vi "SaveIniRegExtSession.vi"(8 "error in (no error)":errorcluster, 11 "RegExt":T1) -> (0 "error out":errorcluster)   [LabVIEW 2014, in "application.lvclass"]
uses:
  application.lvclass
  control/DEF-RegExt.ctl
  <vilib>/Utility/config.llb/NI_LVConfig.lvlib
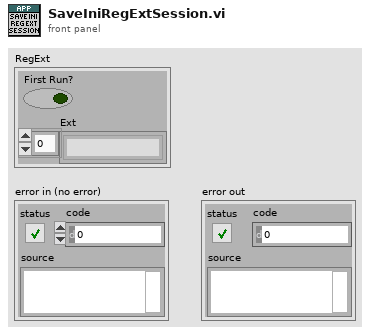
[diagram p1: front panel]
types:
  T1 = typedef "application.lvclass/DEF-RegExt.ctl" = cluster{"First Run?":bool, "Ext":string[]}
  T2 = typedef "NI_LVConfig.lvlib/Config Data RefNum.ctl" = refnum<k1>
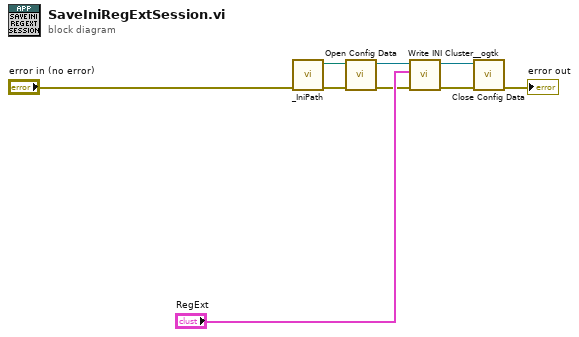
[diagram p0: block diagram]
diagram:
  n1 = call "_IniPath.vi"() -> ("INI Path"=w8:path)  [unwired: 11 in]
  n2 = call <vilib>:"Open Config Data.vi"("error in (no error)"="error in (no error)", "configuration file path"=w8) -> ("error out"=w1:errorcluster, "refnum"=w2:T2)  [unwired: 7 in, 1 out]
  n3 = call <userlib>:"Write INI Cluster__ogtk.vi"("error in (no error)"=w1, "INI Fomatted Cluster"="RegExt", "refnum"=w2) -> ("error out"=w5:errorcluster, "dup refnum"=w4:T2)  [unwired: 7 in]
  n4 = call <vilib>:"Close Config Data.vi"("error in (no error)"=w5, "refnum"=w4) -> ("error out"=→"error out":errorcluster)  [unwired: 8 in, 1 out]
